vi "RD_3_data.vi"(5 "index (row)":i32, 7 "Data array":sgl[][](array[numeric]), 8 "Limit":dbl=0.7 format="%#_13g", 9 "Match_Score":dbl, 10 "name":string="123.txt", 11 "base path":path) -> (1 "output array":sgl[][](array[numeric]), 2 "path":path)   [LabVIEW 2019]
uses:
  <vilib>/regexp/Match Regular Expression.xnode
panel:
  out "Numeric":i32
  out "text":string
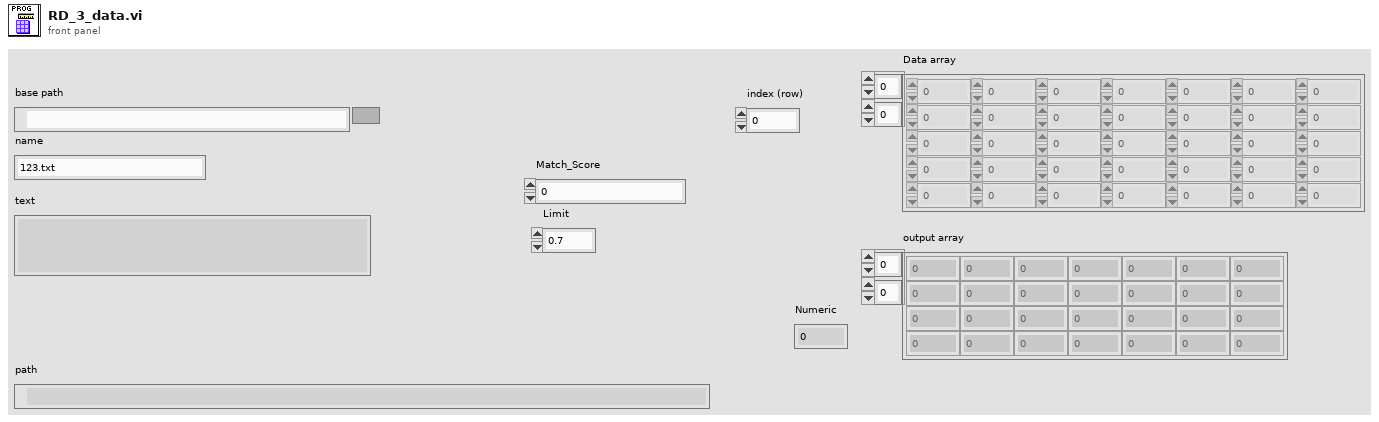
[diagram p1: front panel]
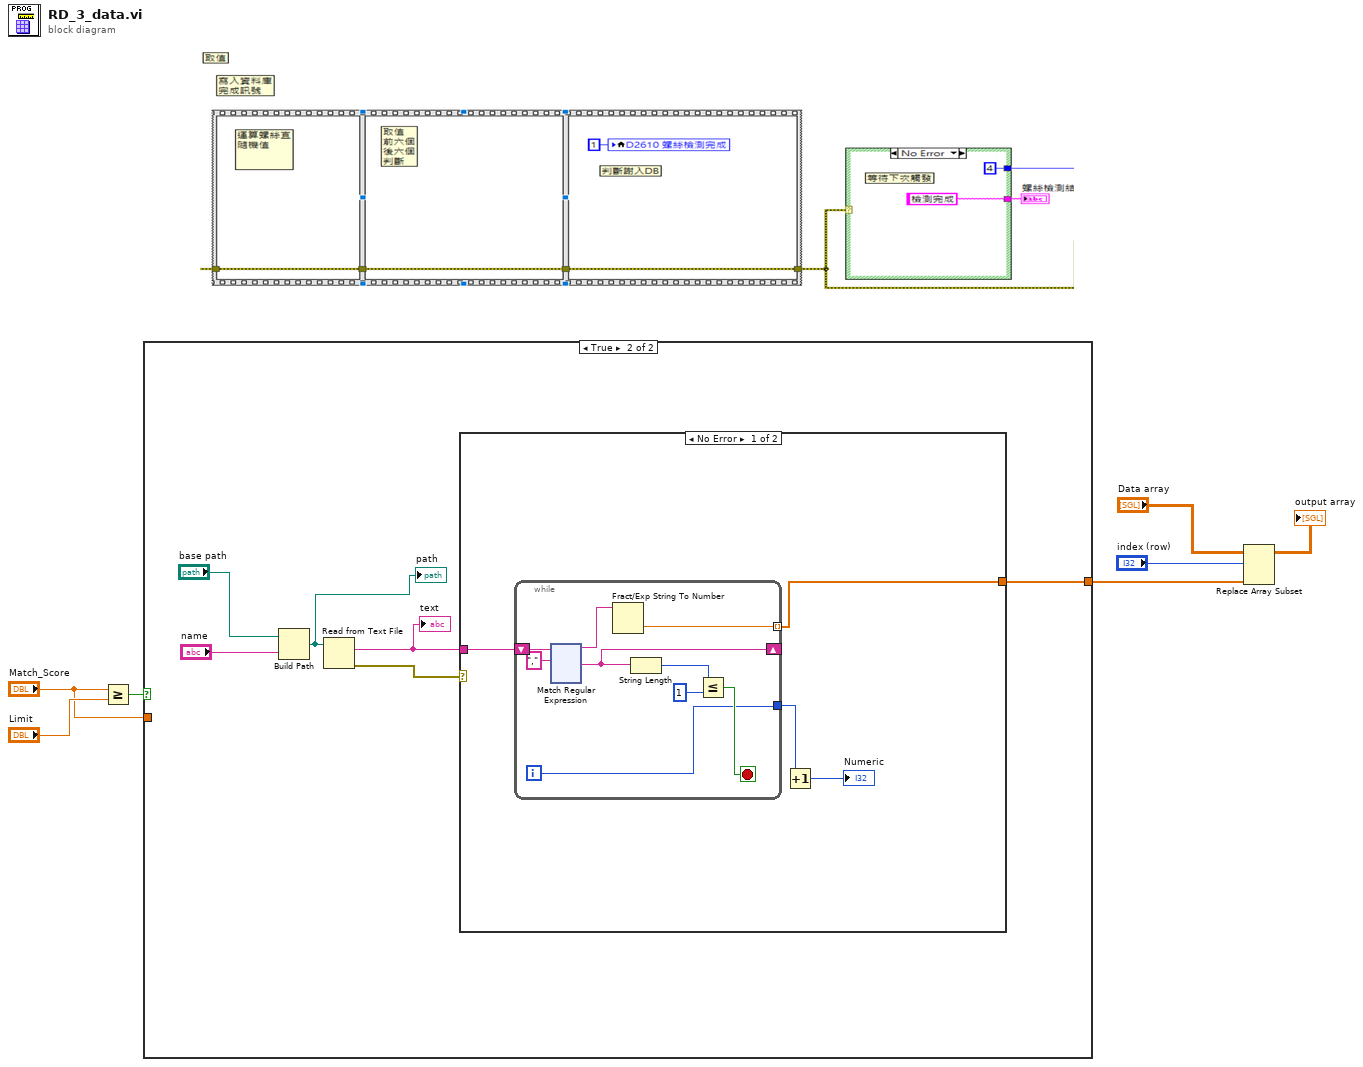
[diagram p0: block diagram]
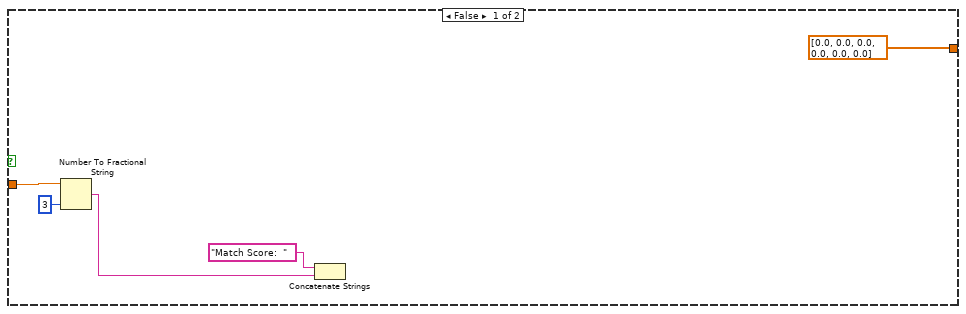
[diagram p2: hidden frame]
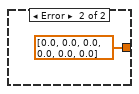
[diagram p3: hidden frame]
diagram:
  n1 = Greater Or Equal?(x="Match_Score", y="Limit") -> (x >= y?=w6:bool)
  n2 = case shown="True" w6 {
    tunnel: "Match_Score" -> [w12 _]
    tunnel: [dbl[] [0.0, 0.0, 0.0, 0.0, 0.0, 0.0] w16] -> w2
    frame False {
      n3 = Number To Fractional String(number=w12, precision (6)=i16 3) -> (F-format string=w9:string)  [unwired: 2 in]
      n4 = Concatenate Strings("Match Score:  ", w9) -> ()  [unwired: 1 out]
    }
    frame True {
      n5 = Build Path(base path="base path", name or relative path="name") -> (appended path=w13:path)
      "path" <- w13
      n6 = Read from Text File(file (use dialog)=w13) -> (text=w17:string, error out=w18:errorcluster)  [unwired: 3 in, 2 out]
      "text" <- w17
      n7 = case shown="No Error" w18 {
        tunnel: w17 -> [w22 _]
        tunnel: [w19 dbl[] [0.0, 0.0, 0.0, 0.0, 0.0, 0.0]] -> w16
        frame No Error {
          n8 = while {
            shift-right: [w24] -> _
            shift-left: w22 -> [w30]
            tunnel: [w25] -> w21
            tunnel: [w23] -> w19 mode=indexing
            i -> [w25]
            stop <- w26 stop-if-true
            n9 = xnode "Match Regular Expression"("input string"=w30, "regular expression"=",") -> ("before match"=w29:string, "after match"=w24:string)  [unwired: 4 in, 3 out]
            n10 = Fract/Exp String To Number(string=w29) -> (number=w23:dbl)  [unwired: 3 in, 1 out]
            n11 = String Length(string=w24) -> (length=w28:i32)
            n12 = Less Or Equal?(x=w28, y=1) -> (x <= y?=w26:bool)
          }
          n13 = Increment(x=w21) -> (x+1=→"Numeric":i32)
        }
        frame Error {
        }
      }
    }
  }
  n14 = Replace Array Subset(array="Data array", new element=w2, index (row)="index (row)") -> (→"output array":sgl[][])  [unwired: 1 in]
